vi "Update.vi"(8 "error in (no error)":errorcluster, 10 "Message in":refnum<class "UpdateMessage.lvclass">, 11 "Galvo in":refnum<class "ImagingModeSPIM.lvclass">) -> (0 "error out":errorcluster, 3 "Galvo out":refnum<class "ImagingModeSPIM.lvclass">)   [LabVIEW 2012, in "ImagingModeSPIM.lvclass"]
doc: "The update method processes the command 'update'. \n\nThe command 'update' is used for receiving new values to be set to the private data of the class. This could be seen as a public set method for setting new parameters to the private class data."
uses:
  ImagingModeSPIM.lvclass
  <vilib>/Distrio/Murmex/UpdateMessage/UpdateMessage.lvclass
  ImagingModeSPIM.lvclass/ImagingModeSPIM.ctl
  Controls/wavelength_ring.ctl
  <vilib>/Distrio/Murmex/Murmex/Murmex.lvclass
panel:
  # "This method is called when the UPDATE\ntrigger is sent. \n\nOverride this method when your component needs to\nrespond to this trigger. \n\nCall parent for proper implementation"
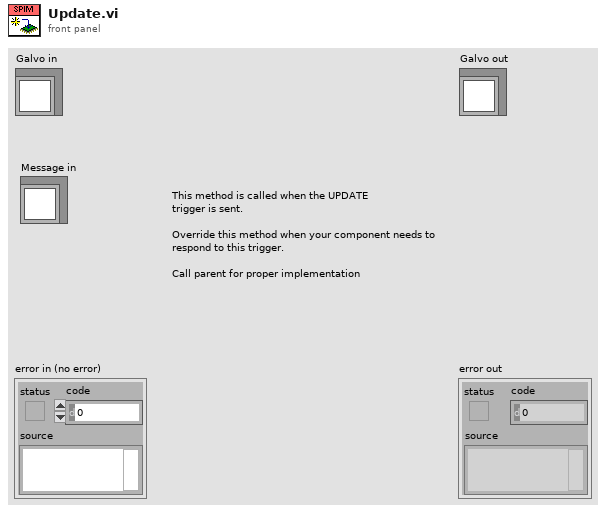
[diagram p1: front panel]
types:
  T1 = typedef "ImagingModeSPIM.lvclass/wavelength_ring.ctl" = dbl
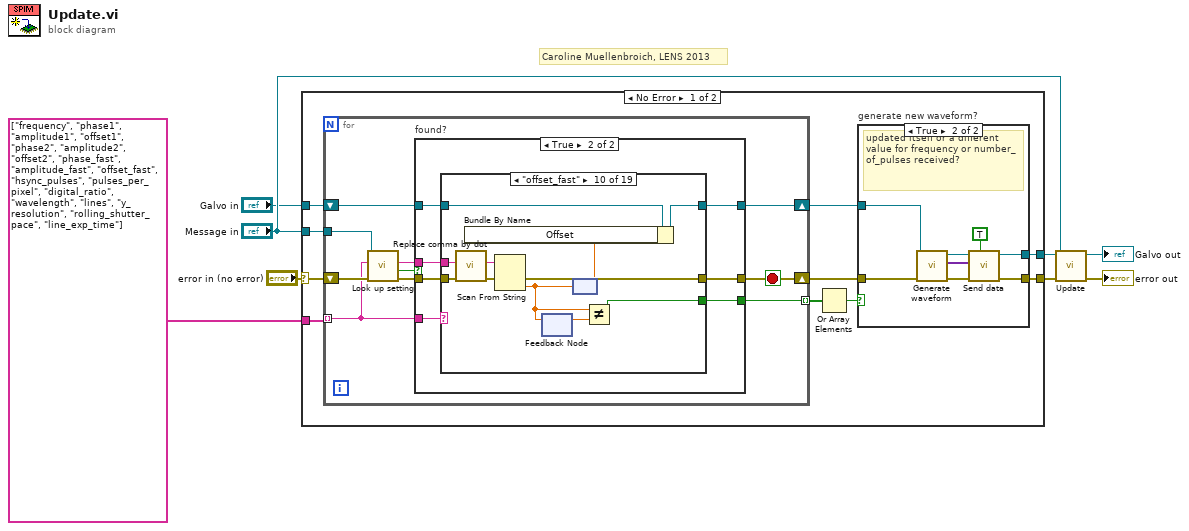
[diagram p0: block diagram]
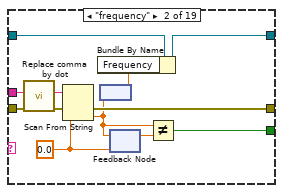
[diagram p5: hidden frame]
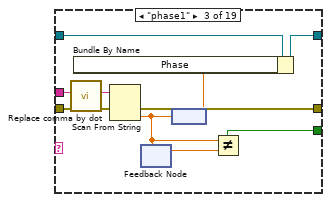
[diagram p6: hidden frame]
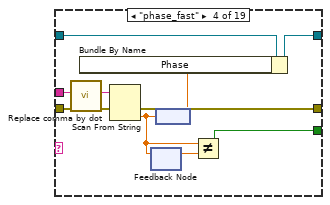
[diagram p7: hidden frame]
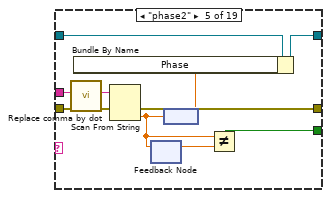
[diagram p8: hidden frame]
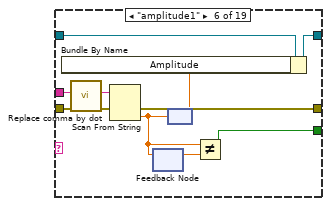
[diagram p9: hidden frame]
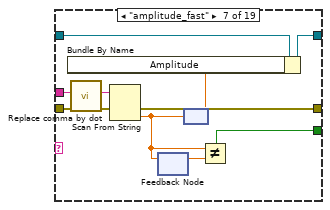
[diagram p10: hidden frame]
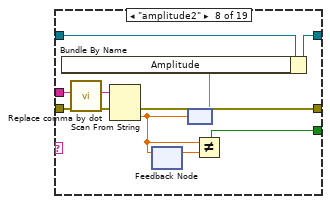
[diagram p11: hidden frame]
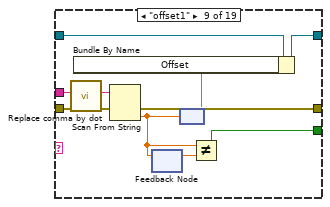
[diagram p12: hidden frame]
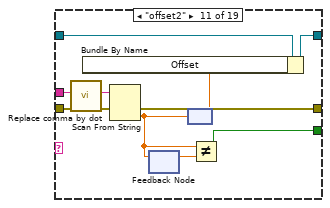
[diagram p13: hidden frame]
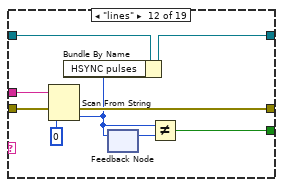
[diagram p14: hidden frame]
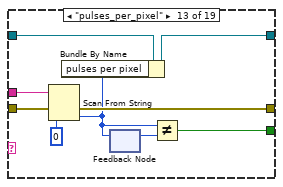
[diagram p15: hidden frame]
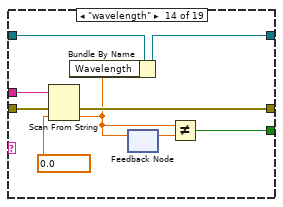
[diagram p16: hidden frame]
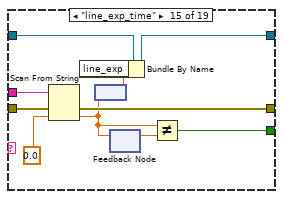
[diagram p17: hidden frame]
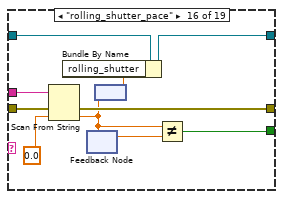
[diagram p18: hidden frame]
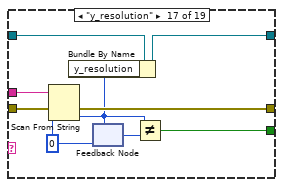
[diagram p19: hidden frame]
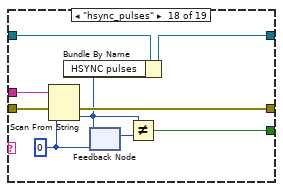
[diagram p20: hidden frame]
diagram:
  # "Caroline Muellenbroich, LENS 2013"
  n1 = case shown="No Error" "error in (no error)" {
    selector: "error in (no error)" -> [w18 w227]
    tunnel: [w13 w228] -> w5
    tunnel: "Galvo in" -> [w11 w228]
    tunnel: [w12 w227] -> w4
    tunnel: "Message in" -> [w17 _]
    tunnel: string[] ["frequency", "phase1", "amplitude1", "offset1", "phase2", "amplitude2", "offset2", "phase_fast", "amplitude_fast", "offset_fast", "hsync_pulses", "pulses_per_pixel", "digital_ratio", "wavelength", "lines", "y_resolution", "rolling_shutter_pace", "line_exp_time"] ("key chains") -> [w14 _]
    frame No Error {
      n2 = for {
        tunnel: w17 -> [w37]
        tunnel: w14 -> [w30] mode=indexing
        shift-right: [w31] -> w16
        shift-left: w18 -> [w38]
        shift-right: [w33] -> w15
        shift-left: w11 -> [w34]
        tunnel: [w29] -> w10 mode=indexing
        stop <- w31 stop-if-true
        n3 = call <vilib>:"Look up setting.vi"("error in (no error)"=w38, "tag name"=w30, "UpdateMessage in"=w37) -> ("error out"=w35:errorcluster, "found?"=w36:bool, "value"=w32:string)  [unwired: 5 in, 1 out]
        n4 = case "found?" shown="True" w36 {
          selector: w36 -> [w39 _]
          tunnel: w35 -> [w41 w46]
          tunnel: [w41 w47] -> w31
          tunnel: w34 -> [w40 w44]
          tunnel: [w40 w45] -> w33
          tunnel: w32 -> [_ w43]
          tunnel: w30 -> [_ w48]
          tunnel: [w39 w42] -> w29
          frame False {
          }
          frame True {
            n5 = case shown="\"offset_fast\"" w48 {
              tunnel: w43 -> [_ w60 w70 w80 w90 w100 w110 w120 w130 w140 w150 w156 w165 w174 w184 w194 w203 w212 w225]
              tunnel: [w50 w58 w68 w78 w88 w98 w108 w118 w128 w138 w148 w157 w166 w175 w185 w195 w204 w213 w223] -> w47
              tunnel: w46 -> [w50 w61 w71 w81 w91 w101 w111 w121 w131 w141 w151 w158 w167 w176 w186 w196 w205 w214 w226]
              tunnel: [w49 w57 w66 w76 w86 w96 w106 w116 w126 w136 w146 w159 w168 w177 w187 w197 w206 w215 w222] -> w45
              tunnel: w44 -> [w49 w59 w69 w79 w89 w99 w109 w119 w129 w139 w149 w160 w169 w178 w188 w198 w207 w216 w224]
              tunnel: [_ w51 w62 w72 w82 w92 w102 w112 w122 w132 w142 w152 w161 w170 w179 w189 w199 w208 w220] -> w42
              frame Default {
              }
              frame "frequency" {
                w53 = 0.0 ("default value 1")
                n6 = call <vilib>:"Replace comma by dot.vi"("input string"=w60) -> ("result string"=w56:string)  [unwired: 10 in]
                n7 = Scan From String(input string=w56, error in=w61, default 1=w53) -> (error out=w58:errorcluster, output 1=w52:dbl)  [unwired: 2 in, 2 out]
                n8 = node(w52) -> (w55:dbl[unit])
                n9 = Bundle By Name(cluster=w59, "Frequency"=w55) -> (w57:refnum<class "ImagingModeSPIM.lvclass">)
                n10 = feedback #1(w53) -> (w54:dbl)
                n11 = feedback-in #1(w52) -> ()
                n12 = Not Equal?(x=w52, y=w54) -> (x != y?=w51:bool)
              }
              frame "phase1" {
                n13 = call <vilib>:"Replace comma by dot.vi"("input string"=w70) -> ("result string"=w65:string)  [unwired: 10 in]
                n14 = Scan From String(input string=w65, error in=w71) -> (error out=w68:errorcluster, output 1=w64:dbl)  [unwired: 3 in, 2 out]
                n15 = feedback #2() -> (w63:dbl)  [unwired: 1 in]
                n16 = feedback-in #2(w64) -> ()
                n17 = node(w64) -> (w67:dbl[unit])
                n18 = Bundle By Name(cluster=w69, "Phase"=w67) -> (w66:refnum<class "ImagingModeSPIM.lvclass">)
                n19 = Not Equal?(x=w64, y=w63) -> (x != y?=w62:bool)
              }
              frame "phase_fast" {
                n20 = call <vilib>:"Replace comma by dot.vi"("input string"=w80) -> ("result string"=w75:string)  [unwired: 10 in]
                n21 = Scan From String(input string=w75, error in=w81) -> (error out=w78:errorcluster, output 1=w73:dbl)  [unwired: 3 in, 2 out]
                n22 = feedback #3() -> (w74:dbl)  [unwired: 1 in]
                n23 = feedback-in #3(w73) -> ()
                n24 = node(w73) -> (w77:dbl[unit])
                n25 = Bundle By Name(cluster=w79, "Phase"=w77) -> (w76:refnum<class "ImagingModeSPIM.lvclass">)
                n26 = Not Equal?(x=w73, y=w74) -> (x != y?=w72:bool)
              }
              frame "phase2" {
                n27 = call <vilib>:"Replace comma by dot.vi"("input string"=w90) -> ("result string"=w85:string)  [unwired: 10 in]
                n28 = Scan From String(input string=w85, error in=w91) -> (error out=w88:errorcluster, output 1=w83:dbl)  [unwired: 3 in, 2 out]
                n29 = feedback #4() -> (w84:dbl)  [unwired: 1 in]
                n30 = feedback-in #4(w83) -> ()
                n31 = node(w83) -> (w87:dbl[unit])
                n32 = Bundle By Name(cluster=w89, "Phase"=w87) -> (w86:refnum<class "ImagingModeSPIM.lvclass">)
                n33 = Not Equal?(x=w83, y=w84) -> (x != y?=w82:bool)
              }
              frame "amplitude1" {
                n34 = call <vilib>:"Replace comma by dot.vi"("input string"=w100) -> ("result string"=w95:string)  [unwired: 10 in]
                n35 = Scan From String(input string=w95, error in=w101) -> (error out=w98:errorcluster, output 1=w94:dbl)  [unwired: 3 in, 2 out]
                n36 = feedback #5() -> (w93:dbl)  [unwired: 1 in]
                n37 = feedback-in #5(w94) -> ()
                n38 = node(w94) -> (w97:dbl[unit])
                n39 = Bundle By Name(cluster=w99, "Amplitude"=w97) -> (w96:refnum<class "ImagingModeSPIM.lvclass">)
                n40 = Not Equal?(x=w94, y=w93) -> (x != y?=w92:bool)
              }
              frame "amplitude_fast" {
                n41 = call <vilib>:"Replace comma by dot.vi"("input string"=w110) -> ("result string"=w105:string)  [unwired: 10 in]
                n42 = Scan From String(input string=w105, error in=w111) -> (error out=w108:errorcluster, output 1=w104:dbl)  [unwired: 3 in, 2 out]
                n43 = feedback #6() -> (w103:dbl)  [unwired: 1 in]
                n44 = feedback-in #6(w104) -> ()
                n45 = node(w104) -> (w107:dbl[unit])
                n46 = Bundle By Name(cluster=w109, "Amplitude"=w107) -> (w106:refnum<class "ImagingModeSPIM.lvclass">)
                n47 = Not Equal?(x=w104, y=w103) -> (x != y?=w102:bool)
              }
              frame "amplitude2" {
                n48 = call <vilib>:"Replace comma by dot.vi"("input string"=w120) -> ("result string"=w115:string)  [unwired: 10 in]
                n49 = Scan From String(input string=w115, error in=w121) -> (error out=w118:errorcluster, output 1=w113:dbl)  [unwired: 3 in, 2 out]
                n50 = feedback #7() -> (w114:dbl)  [unwired: 1 in]
                n51 = feedback-in #7(w113) -> ()
                n52 = node(w113) -> (w117:dbl[unit])
                n53 = Bundle By Name(cluster=w119, "Amplitude"=w117) -> (w116:refnum<class "ImagingModeSPIM.lvclass">)
                n54 = Not Equal?(x=w113, y=w114) -> (x != y?=w112:bool)
              }
              frame "offset1" {
                n55 = call <vilib>:"Replace comma by dot.vi"("input string"=w130) -> ("result string"=w125:string)  [unwired: 10 in]
                n56 = Scan From String(input string=w125, error in=w131) -> (error out=w128:errorcluster, output 1=w123:dbl)  [unwired: 3 in, 2 out]
                n57 = feedback #8() -> (w124:dbl)  [unwired: 1 in]
                n58 = feedback-in #8(w123) -> ()
                n59 = node(w123) -> (w127:dbl[unit])
                n60 = Bundle By Name(cluster=w129, "Offset"=w127) -> (w126:refnum<class "ImagingModeSPIM.lvclass">)
                n61 = Not Equal?(x=w123, y=w124) -> (x != y?=w122:bool)
              }
              frame "offset_fast" {
                n62 = call <vilib>:"Replace comma by dot.vi"("input string"=w140) -> ("result string"=w135:string)  [unwired: 10 in]
                n63 = Scan From String(input string=w135, error in=w141) -> (error out=w138:errorcluster, output 1=w134:dbl)  [unwired: 3 in, 2 out]
                n64 = feedback #9() -> (w133:dbl)  [unwired: 1 in]
                n65 = feedback-in #9(w134) -> ()
                n66 = node(w134) -> (w137:dbl[unit])
                n67 = Bundle By Name(cluster=w139, "Offset"=w137) -> (w136:refnum<class "ImagingModeSPIM.lvclass">)
                n68 = Not Equal?(x=w134, y=w133) -> (x != y?=w132:bool)
              }
              frame "offset2" {
                n69 = call <vilib>:"Replace comma by dot.vi"("input string"=w150) -> ("result string"=w145:string)  [unwired: 10 in]
                n70 = Scan From String(input string=w145, error in=w151) -> (error out=w148:errorcluster, output 1=w143:dbl)  [unwired: 3 in, 2 out]
                n71 = feedback #10() -> (w144:dbl)  [unwired: 1 in]
                n72 = feedback-in #10(w143) -> ()
                n73 = node(w143) -> (w147:dbl[unit])
                n74 = Bundle By Name(cluster=w149, "Offset"=w147) -> (w146:refnum<class "ImagingModeSPIM.lvclass">)
                n75 = Not Equal?(x=w143, y=w144) -> (x != y?=w142:bool)
              }
              frame "lines" {
                n76 = Scan From String(input string=w156, error in=w158, default 1=0) -> (error out=w157:errorcluster, output 1=w153:i32)  [unwired: 2 in, 2 out]
                n77 = Bundle By Name(cluster=w160, "HSYNC pulses"=w153) -> (w159:refnum<class "ImagingModeSPIM.lvclass">)
                n78 = feedback #11() -> (w154:i32)  [unwired: 1 in]
                n79 = feedback-in #11(w153) -> ()
                n80 = Not Equal?(x=w153, y=w154) -> (x != y?=w152:bool)
              }
              frame "pulses_per_pixel" {
                n81 = Scan From String(input string=w165, error in=w167, default 1=0) -> (error out=w166:errorcluster, output 1=w162:i32)  [unwired: 2 in, 2 out]
                n82 = Bundle By Name(cluster=w169, "pulses per pixel"=w162) -> (w168:refnum<class "ImagingModeSPIM.lvclass">)
                n83 = feedback #12() -> (w163:i32)  [unwired: 1 in]
                n84 = feedback-in #12(w162) -> ()
                n85 = Not Equal?(x=w162, y=w163) -> (x != y?=w161:bool)
              }
              frame "wavelength" {
                w173 = T1 0.0 items=["405nm"=0.0, "445nm"=0.1, "491nm"=0.27, "515nm"=0.22, "561nm"=0.3] ("settings.Wavelength")
                n86 = Scan From String(input string=w174, error in=w176, default 1=w173) -> (error out=w175:errorcluster, output 1=w171:T1)  [unwired: 2 in, 2 out]
                n87 = Bundle By Name(cluster=w178, "Wavelength"=w171) -> (w177:refnum<class "ImagingModeSPIM.lvclass">)
                n88 = feedback #13() -> (w172:T1)  [unwired: 1 in]
                n89 = feedback-in #13(w171) -> ()
                n90 = Not Equal?(x=w171, y=w172) -> (x != y?=w170:bool)
              }
              frame "line_exp_time" {
                n91 = Scan From String(input string=w184, error in=w186, default 1=0.0) -> (error out=w185:errorcluster, output 1=w180:dbl)  [unwired: 2 in, 2 out]
                n92 = node(w180) -> (w183:dbl[unit])
                n93 = Bundle By Name(cluster=w188, "line_exp"=w183) -> (w187:refnum<class "ImagingModeSPIM.lvclass">)
                n94 = feedback #14() -> (w181:dbl)  [unwired: 1 in]
                n95 = feedback-in #14(w180) -> ()
                n96 = Not Equal?(x=w180, y=w181) -> (x != y?=w179:bool)
              }
              frame "rolling_shutter_pace" {
                n97 = Scan From String(input string=w194, error in=w196, default 1=0.0) -> (error out=w195:errorcluster, output 1=w190:dbl)  [unwired: 2 in, 2 out]
                n98 = feedback #15() -> (w191:dbl)  [unwired: 1 in]
                n99 = feedback-in #15(w190) -> ()
                n100 = node(w190) -> (w193:dbl[unit])
                n101 = Bundle By Name(cluster=w198, "rolling_shutter"=w193) -> (w197:refnum<class "ImagingModeSPIM.lvclass">)
                n102 = Not Equal?(x=w190, y=w191) -> (x != y?=w189:bool)
              }
              frame "y_resolution" {
                w200 = 0
                n103 = Scan From String(input string=w203, error in=w205, default 1=w200) -> (error out=w204:errorcluster, output 1=w201:i32)  [unwired: 2 in, 2 out]
                n104 = Bundle By Name(cluster=w207, "y_resolution"=w201) -> (w206:refnum<class "ImagingModeSPIM.lvclass">)
                n105 = feedback #16(w200) -> (w202:i32)
                n106 = feedback-in #16(w201) -> ()
                n107 = Not Equal?(x=w201, y=w202) -> (x != y?=w199:bool)
              }
              frame "hsync_pulses" {
                w209 = 0
                n108 = Scan From String(input string=w212, error in=w214, default 1=w209) -> (error out=w213:errorcluster, output 1=w211:i32)  [unwired: 2 in, 2 out]
                n109 = Bundle By Name(cluster=w216, "HSYNC pulses"=w211) -> (w215:refnum<class "ImagingModeSPIM.lvclass">)
                n110 = feedback-in #17(w211) -> ()
                n111 = feedback #17(w209) -> (w210:i32)
                n112 = Not Equal?(x=w211, y=w210) -> (x != y?=w208:bool)
              }
              frame "digital_ratio" {
                w217 = 0.0 ("default value 1")
                n113 = call <vilib>:"Replace comma by dot.vi"("input string"=w225) -> ("result string"=w221:string)  [unwired: 10 in]
                n114 = Scan From String(input string=w221, error in=w226, default 1=w217) -> (error out=w223:errorcluster, output 1=w218:dbl)  [unwired: 2 in, 2 out]
                n115 = Bundle By Name(cluster=w224, "digital ratio"=w218) -> (w222:refnum<class "ImagingModeSPIM.lvclass">)
                n116 = feedback #18(w217) -> (w219:dbl)
                n117 = feedback-in #18(w218) -> ()
                n118 = Not Equal?(x=w218, y=w219) -> (x != y?=w220:bool)
              }
            }
          }
        }
      }
      n119 = Or Array Elements(Boolean array=w10) -> (logical OR=w9:bool)
      n120 = case "generate new waveform?" shown="True" w9 {
        tunnel: w16 -> [w19 w28]
        tunnel: w15 -> [w20 w27]
        tunnel: [w20 w26] -> w13
        tunnel: [w19 w25] -> w12
        frame False {
        }
        frame True {
          # "updated itself or a different value for frequency or number_of_pulses received?"
          n121 = call-dynamic "Generate waveform.vi"("error in (no error)"=w28, "Galvo in"=w27) -> ("error out"=w23:errorcluster, "Array"=w21:variant[], "Galvo out"=w22:refnum<class "ImagingModeSPIM.lvclass">)  [unwired: 7 in]
          n122 = call <vilib>:"Send data.vi"("is finalised data? (T)"=TRUE, "error in (no error)"=w23, "data (channels array)"=w21, "Murmex in"=w22) -> ("error out"=w25:errorcluster, "Murmex out"=w26:refnum<class "ImagingModeSPIM.lvclass">)  [unwired: 6 in]
        }
      }
    }
    frame Error {
    }
  }
  n123 = call-parent "Update.vi"("error in (no error)"=w4, "Message in"="Message in", "Murmex in"=w5) -> ("error out"=→"error out":errorcluster, "Murmex out"=→"Galvo out":refnum<class "ImagingModeSPIM.lvclass">)  [unwired: 7 in]
